vi "DeInit.vi"(8 "error in (no error)":errorcluster, 11 "HRS_Spectrometer in":refnum<class "HRS_Spectrometer.lvclass">) -> (0 "error out":errorcluster, 3 "HRS_Spectrometer out":refnum<class "HRS_Spectrometer.lvclass">)   [LabVIEW 2023, in "Spectrometer Library.lvlib" / "HRS_Spectrometer.lvlib" / "HRS_Spectrometer.lvclass"]
uses:
  HRS_Spectrometer.lvclass
  <vilib>/Instr/_visa.llb/Select Event Type.ctl
  HRS_Spectrometer.lvclass/HRS_Spectrometer.ctl
  <vilib>/ActorFramework/Message Enqueuer/Message Enqueuer.lvclass/Message Enqueuer.ctl
  <vilib>/ActorFramework/Message Enqueuer/Enqueue.vi
  <vilib>/ActorFramework/Stop Msg/Stop Msg.lvclass
  <vilib>/ActorFramework/Message Priority Queue/Priority Enqueue.vi
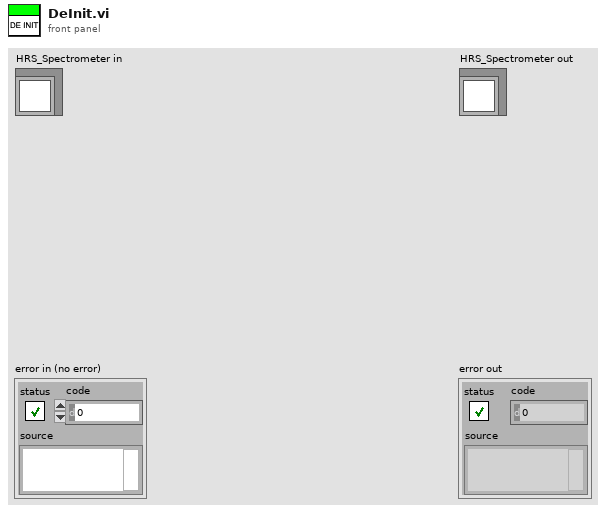
[diagram p1: front panel]
types:
  T1 = typedef "Select Event Type.ctl" = u32
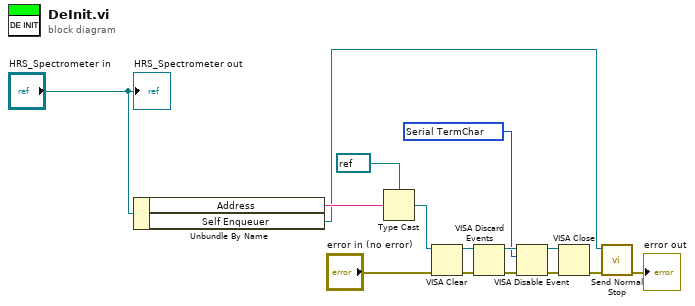
[diagram p0: block diagram]
diagram:
  w7 = T1 1073684516 items=["Service Request"=1073684491, "Trigger"=3221168138, "Clear"=1073684493, "VXI Signal"=1073684512, "VXI/VME Interrupt"=3221168161, "VXI/VME Sysfail"=1073684509, "VXI/VME Sysreset"=1073684510, "GPIB CIC"=1073684498, "GPIB Talk"=1073684499, "GPIB Listen"=1073684500, "PXI Interrupt"=1073684514, "Serial Break"=1073684515, "Serial TermChar"=1073684516, "Serial CTS"=1073684521, "Serial DSR"=1073684522, "Serial DCD"=1073684524, "Serial RI"=1073684526, "Serial Character"=1073684533, "USB Interrupt"=1073684535, "All Enabled"=1073709055] ("Event Type")
  n1 = Unbundle By Name("HRS_Spectrometer in") -> ("Address"=w5:string, "Self Enqueuer"=w3:refnum<class "Message Enqueuer.lvclass">)
  n2 = Type Cast(type=refnum<visa-resource-name> refnum ("VISA resource name"), x=w5) -> (*(type *) &x=w4:refnum<visa-resource-name>)
  n3 = VISA Clear(VISA resource name=w4, error in (no error)="error in (no error)") -> (VISA resource name out=w11:refnum<visa-resource-name>, error out=w9:errorcluster)
  n4 = VISA Discard Events(8:w9, 11:w11) -> (0:w12:errorcluster, 3:w13:refnum<visa-resource-name>)  [unwired: 2 in]
  n5 = VISA Disable Event(8:w12, 10:w7, 11:w13) -> (0:w8:errorcluster, 3:w10:refnum<visa-resource-name>)  [unwired: 1 in]
  n6 = VISA Close(VISA resource name=w10, error in (no error)=w8) -> (error out=w2:errorcluster)
  n7 = call <vilib>:"Send Normal Stop.vi"("error in (no error)"=w2, "Message Enqueuer"=w3) -> ("error out"=→"error out":errorcluster)  [unwired: 9 in]
  "HRS_Spectrometer out" <- "HRS_Spectrometer in"
